vi "lab3.vi"() -> ()   [LabVIEW 2020]
panel:
  out "D":dbl[][](array[numeric])
  out "С":dbl[][](array[numeric])
  out "B":dbl[][](array[numeric])
  out "A":dbl[][](array[numeric])
  in  "Col":dbl
  in  "Lines":dbl
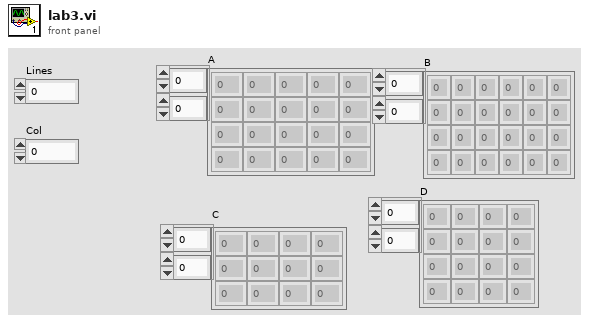
[diagram p1: front panel]
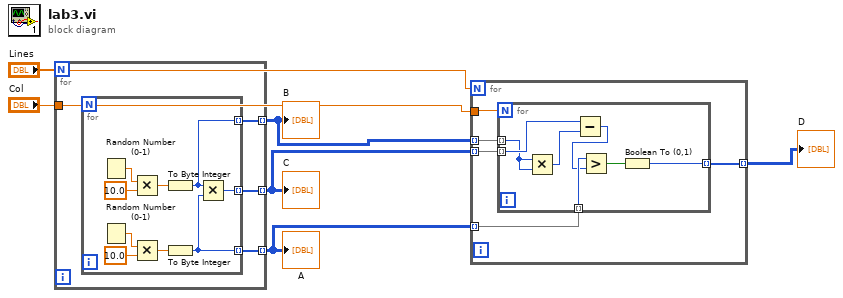
[diagram p0: block diagram]
diagram:
  n1 = for {
    N: "Lines" -> [_]
    tunnel: "Col" -> [w10]
    tunnel: [w9] -> w3 mode=indexing
    tunnel: [w8] -> w2 mode=indexing
    tunnel: [w7] -> w4 mode=indexing
    n2 = for {
      N: w10 -> [_]
      tunnel: [w13] -> w9 mode=indexing
      tunnel: [w12] -> w8 mode=indexing
      tunnel: [w11] -> w7 mode=indexing
      n3 = Random Number (0-1)() -> (number: 0 to 1=w19:dbl)
      n4 = Random Number (0-1)() -> (number: 0 to 1=w17:dbl)
      n5 = Multiply(x=w19, y=10.0) -> (x*y=w15:dbl)
      n6 = Multiply(x=w17, y=10.0) -> (x*y=w14:dbl)
      n7 = To Byte Integer(number=w15) -> (8bit integer=w13:i8)
      n8 = To Byte Integer(number=w14) -> (8bit integer=w12:i8)
      n9 = Multiply(x=w13, y=w12) -> (x*y=w11:i8)
    }
  }
  "B" <- w3
  "A" <- w2
  "С" <- w4
  n10 = for {
    N: "Lines" -> [_]
    tunnel: "Col" -> [w24]
    tunnel: w4 -> [w23] mode=indexing
    tunnel: w3 -> [w22] mode=indexing
    tunnel: w2 -> [w21] mode=indexing
    tunnel: [w20] -> w1 mode=indexing
    n11 = for {
      N: w24 -> [_]
      tunnel: w23 -> [w31] mode=indexing
      tunnel: w22 -> [w27] mode=indexing
      tunnel: w21 -> [w28] mode=indexing
      tunnel: [w29] -> w20 mode=indexing
      n12 = Multiply(x=w27, y=w27) -> (x*y=w26:i8)
      n13 = Subtract(x=w31, y=w26) -> (x-y=w25:i8)
      n14 = Greater?(x=w28, y=w25) -> (0:w30:bool)
      n15 = Boolean To (0,1)(Boolean=w30) -> (0, 1=w29:i16)
    }
  }
  "D" <- w1
